vi "Start Task-Points.vi"(8 "error in":errorcluster, 10 "Task Ident":string, 11 "Series Actor in":refnum<class "Series Actor.lvclass">) -> (0 "error out":errorcluster, 3 "Series Actor out":refnum<class "Series Actor.lvclass">)   [LabVIEW 2023, in "Series Actor.lvlib" / "Series Actor.lvclass"]
uses:
  Series Actor.lvclass
  Series Actor.lvclass/Series Actor.ctl
  <vilib>/Utility/error.llb/Error Cluster From Error Code.vi
  <vilib>/ErrorRing/Error Ring.xnode
  Task/ITask Actor/ITask Actor Messages/Start Msg/Start Msg.lvclass
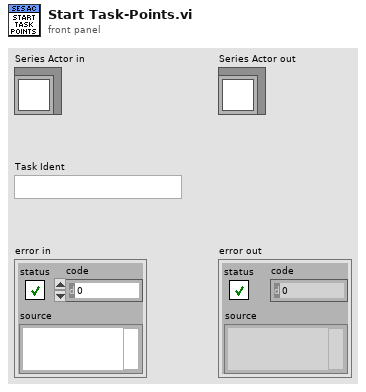
[diagram p1: front panel]
types:
  T1 = map{string, refnum<class "Message Enqueuer.lvclass">}
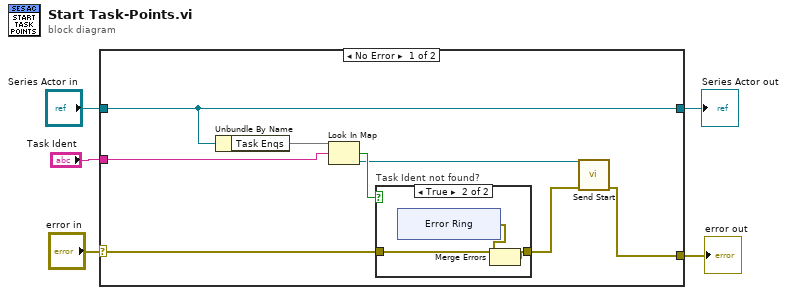
[diagram p0: block diagram]
diagram:
  n1 = case shown="No Error" "error in" {
    selector: "error in" -> [w7 w24]
    tunnel: [w6 w24] -> w4
    tunnel: [w8 w23] -> w2
    tunnel: "Series Actor in" -> [w8 w23]
    tunnel: "Task Ident" -> [w9 _]
    frame No Error {
      n2 = Unbundle By Name(w8) -> ("Task Enqs"=w13:T1)
      n3 = Look In Map(map=w13, key=w9) -> (key not found?=w12:bool, value=w10:refnum<class "Message Enqueuer.lvclass">)  [unwired: 1 in]
      n4 = case "Task Ident not found?" shown="True" w12 {
        tunnel: w7 -> [w14 w17]
        tunnel: [w14 w15] -> w11
        frame False {
        }
        frame True {
          n5 = xnode "Error Ring"() -> ("error out"=w16:errorcluster)
          n6 = Merge Errors(w17, w16) -> (w15:errorcluster)
        }
      }
      n7 = call "Send Start.vi"("error in (no error)"=w11, "Message Enqueuer"=w10) -> ("error out"=w6:errorcluster)  [unwired: 8 in, 1 out]
    }
    frame Error {
    }
  }
  "error out" <- w4
  "Series Actor out" <- w2
